vi "Get PPMS Class.vi"(8 "error in (no error)":errorcluster, 11 "instrument.PPMS":refnum<class "instrument.PPMS.lvclass">) -> (0 "error out":errorcluster, 2 "Select PPMS":T1, 3 "instrument.PPMS out":refnum<class "instrument.PPMS.lvclass">)   [LabVIEW 2019, in "instrument.PPMS.lvclass"]
uses:
  instrument.PPMS.lvclass
  Typedefs/Select PPMS--Enum.ctl
  instrument.PPMS1/instrument.PPMS1.lvclass
  instrument.PPMS2/instrument.PPMS2.lvclass
  instrument.PPMS3/instrument.PPMS3.lvclass
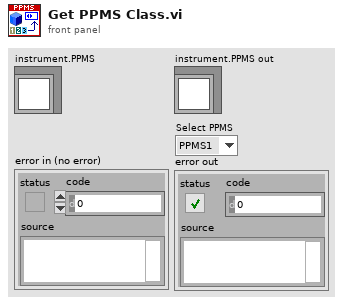
[diagram p1: front panel]
types:
  T1 = typedef "instrument.PPMS.lvclass/Select PPMS--Enum.ctl" = enum16{"PPMS1", "PPMS2", "PPMS3", "simulate"}
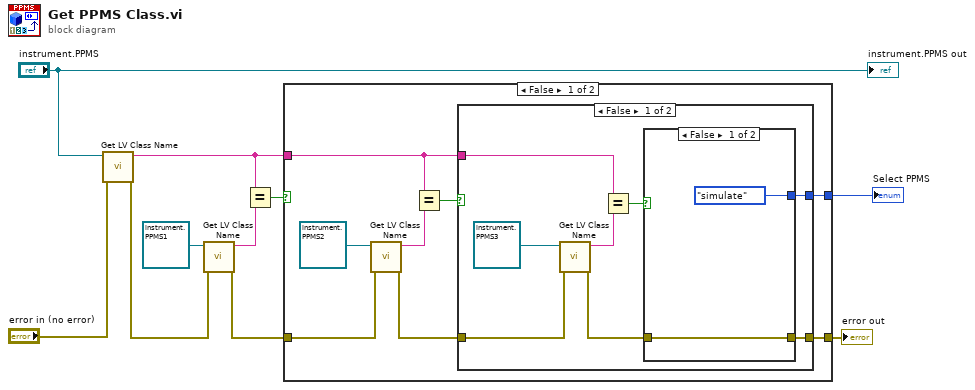
[diagram p0: block diagram]
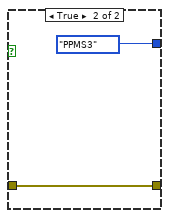
[diagram p2: hidden frame]
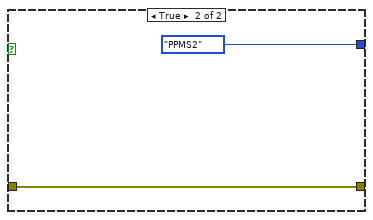
[diagram p3: hidden frame]
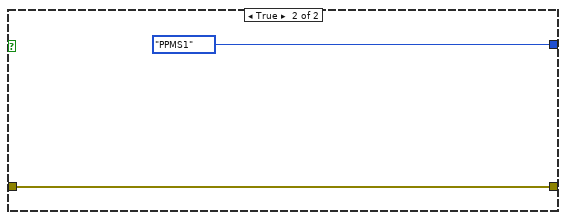
[diagram p4: hidden frame]
diagram:
  n1 = call <vilib>:"Get LV Class Name.vi"("error in (no error)"="error in (no error)", "object"="instrument.PPMS") -> ("error out"=w3:errorcluster, "class name"=w5:string)  [unwired: 8 in]
  n2 = call <vilib>:"Get LV Class Name.vi"("error in (no error)"=w3, "object"=refnum<class "instrument.PPMS1.lvclass"> refnum ("instrument.PPMS1.lvclass")) -> ("error out"=w2:errorcluster, "class name"=w7:string)  [unwired: 8 in]
  n3 = Equal?(x=w5, y=w7) -> (x = y?=w10:bool)
  n4 = case shown="False" w10 {
    tunnel: [w14 Select_PPMS--Enum."PPMS1" ("Select PPMS")] -> w6
    tunnel: w5 -> [w12 _]
    tunnel: w2 -> [w16 w33]
    tunnel: [w11 w33] -> w1
    frame False {
      n5 = call <vilib>:"Get LV Class Name.vi"("error in (no error)"=w16, "object"=refnum<class "instrument.PPMS2.lvclass"> refnum ("instrument.PPMS2.lvclass")) -> ("error out"=w15:errorcluster, "class name"=w18:string)  [unwired: 8 in]
      n6 = Equal?(x=w12, y=w18) -> (x = y?=w17:bool)
      n7 = case shown="False" w17 {
        tunnel: w15 -> [w23 w31]
        tunnel: [w21 Select_PPMS--Enum."PPMS2" ("Select PPMS")] -> w14
        tunnel: w12 -> [w24 _]
        tunnel: [w20 w31] -> w11
        frame False {
          n8 = call <vilib>:"Get LV Class Name.vi"("error in (no error)"=w23, "object"=refnum<class "instrument.PPMS3.lvclass"> refnum ("instrument.PPMS3.lvclass")) -> ("error out"=w19:errorcluster, "class name"=w26:string)  [unwired: 8 in]
          n9 = Equal?(x=w24, y=w26) -> (x = y?=w22:bool)
          n10 = case shown="False" w22 {
            tunnel: [Select_PPMS--Enum."simulate" ("Select PPMS") Select_PPMS--Enum."PPMS3" ("Select PPMS")] -> w21
            tunnel: [w28 w29] -> w20
            tunnel: w19 -> [w28 w29]
            frame False {
            }
            frame True {
            }
          }
        }
        frame True {
        }
      }
    }
    frame True {
    }
  }
  "Select PPMS" <- w6
  "error out" <- w1
  "instrument.PPMS out" <- "instrument.PPMS"
